vi "AddUser.vi"(8 "Group":u8(ring) items=["Operator", "Engineering", "Admin"], 9 "Pwd":string caption="Password:", 10 "User":string caption="User Name:", 11 "UserLibFile":path) -> (2 "Success?":bool)   [LabVIEW 2020]
uses:
  <userlib>/_OpenG.lib/md5/md5.llb/MD5 Message Digest (Hexadecimal String)__ogtk.vi
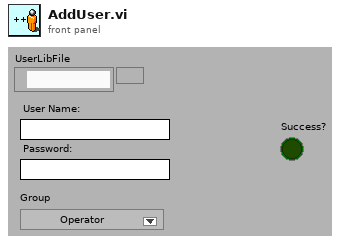
[diagram p1: front panel]
types:
  T1 = enum16{"open", "replace", "create", "open or create", "replace or create", "replace or create with confirmation"}
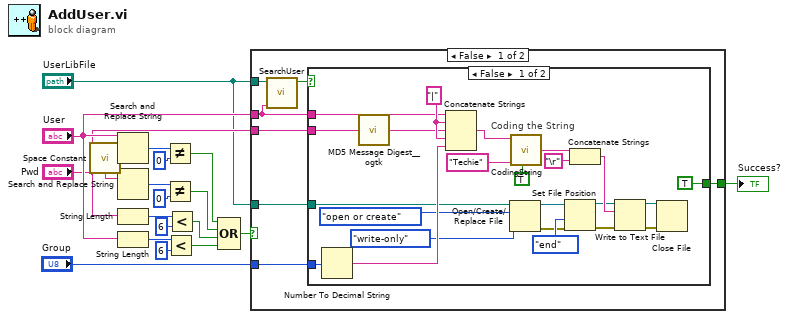
[diagram p0: block diagram]
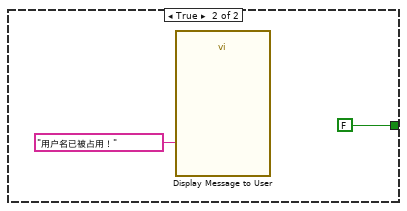
[diagram p2: hidden frame]
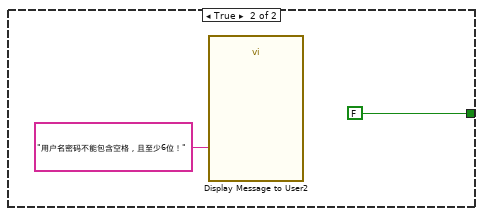
[diagram p3: hidden frame]
diagram:
  n1 = call <vilib>:"Space Constant.vi"() -> ("String"=w18:string)
  n2 = Search and Replace String(input string="User", search string=w18) -> (number of replacements=w14:i32)  [unwired: 2 in, 7 out]
  n3 = Search and Replace String(input string="Pwd", search string=w18) -> (number of replacements=w17:i32)  [unwired: 2 in, 7 out]
  n4 = String Length(string="Pwd") -> (length=w10:i32)
  n5 = String Length(string="User") -> (length=w13:i32)
  n6 = Not Equal?(x=w14, y=0) -> (x != y?=w9:bool)
  n7 = Not Equal?(x=w17, y=0) -> (x != y?=w7:bool)
  n8 = Less?(x=w13, y=6) -> (x < y?=w3:bool)
  n9 = Less?(x=w10, y=6) -> (x < y?=w6:bool)
  n10 = Compound Arithmetic op=OR(w9, w7, w6, w3) -> (w8:bool)
  n11 = case shown="False" w8 {
    tunnel: "User" -> [w22 _]
    tunnel: "Pwd" -> [w26 _]
    tunnel: [w25 FALSE] -> w19
    tunnel: "UserLibFile" -> [w23 _]
    tunnel: "Group" -> [w21 _]
    tunnel: "UserLibFile" -> [w20 _]
    frame False {
      n12 = call "SearchUser.vi"("User"=w22, "UserLibFile"=w23) -> ("Exist?"=w24:bool)  [unwired: 6 in, 3 out]
      n13 = case shown="False" w24 {
        tunnel: w22 -> [w36 _]
        tunnel: w26 -> [w28 _]
        tunnel: [TRUE FALSE] -> w25
        tunnel: w21 -> [w30 _]
        tunnel: w20 -> [w29 _]
        frame False {
          w46 = "|" ("string")
          # "Coding the String"
          n14 = Number To Decimal String(number=w30) -> (decimal integer string=w47:string)  [unwired: 1 out]
          n15 = call-poly <userlib>:"MD5 Message Digest__ogtk.vi"("Message"=w28) -> ("MD5 Message Digest"=w27:string)
          n16 = Concatenate Strings(w36, w46, w27, w46, w47) -> (w34:string)
          n17 = Open/Create/Replace File(file path (use dialog)=w29, operation (0:open)=T1."open or create", access (0:read/write)=enum16{"read/write", "read-only", "write-only"}."write-only") -> (refnum out=w39:refnum<file>, error out=w40:errorcluster)  [unwired: 1 in, 3 out]
          n18 = call "CodingString.vi"("InputStr"=w34, "key"="Techie", "Coding(T)?"=TRUE) -> ("Output"=w33:string)  [unwired: 2 out]
          n19 = Set File Position(refnum=w39, from (0:start)=enum16{"start", "end", "current"}."end", error in=w40) -> (refnum out=w43:refnum<file>, error out=w42:errorcluster)  [unwired: 1 out]
          n20 = Concatenate Strings(w33, "\r") -> (w49:string)
          n21 = Write to Text File(file (use dialog)=w43, text=w49, error in=w42) -> (refnum out=w45:refnum<file>, error out=w44:errorcluster)  [unwired: 2 out]
          n22 = Close File(refnum=w45, error in=w44) -> ()  [unwired: 2 out]
        }
        frame True {
          n23 = call "Display Message to User"("Message"="用户名已被占用！") -> ()  [unwired: 2 in, 9 out]
        }
      }
    }
    frame True {
      n24 = call "Display Message to User2"("Message"="用户名密码不能包含空格，且至少6位！") -> ()  [unwired: 2 in, 9 out]
    }
  }
  "Success?" <- w19
